vi "Test UTF Job.vi"() -> ()   [LabVIEW 2014]
uses:
  Core/LabVIEW CI Service/Extensions/Run UTF/Run UTF/Run UTF - STYP.ctl
  Core/LabVIEW CI Service/Classes/Status Updater/Status Updater.lvclass/Status Updater.ctl
  Core/LabVIEW CI Service/Classes/Job/Job.lvclass/Job.ctl
  Core/LabVIEW CI Service/Extensions/Run UTF/Run UTF/Run UTF.lvclass
  Core/LabVIEW CI Service/Classes/Status Updater/Status Updater.lvclass
  Core/LabVIEW CI Service/Classes/Job/Job.lvclass
panel:
  in  "Workspace Path":path=path "P:/alsmith/Sales/users/ACS/LabVIEW Continuous Integration/Jenkins Sample Project/Run VI Golden DUT.vi"
  out "Results":T1 {"Status" items=["Service Error"=504, "Abort"=503, "Fail"=500, "Pass"=200]}
  out "Steps":string[](array[string])
  out "Progress Percents":u32[](array[numeric])
  in  "VI Path":path=path "P:/alsmith/Sales/users/ACS/LabVIEW Continuous Integration/Jenkins Sample Project/Run VI Golden DUT.vi"
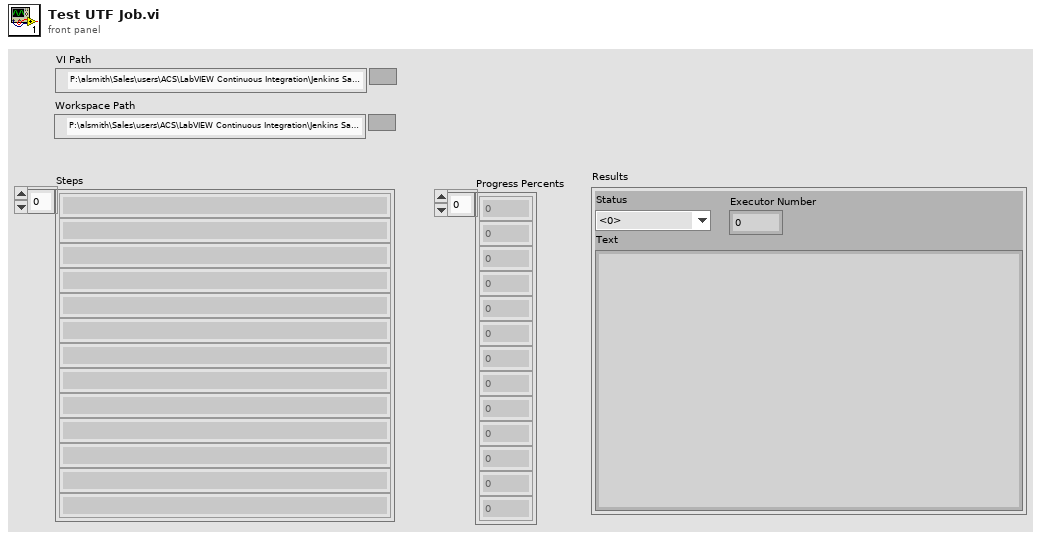
[diagram p1: front panel]
types:
  T1 = cluster{"Status":u16, "Text":string, "Executor Number":i32}
  T2 = typedef "Run UTF - STYP.ctl" = cluster{"Project Path":string}
  T3 = cluster{"Event Registration Refnum":refnum<event-registration>, "Event Registration Refnum":refnum<event-registration>}
  T4 = typedef "Job Results - STYP.ctl" = cluster{"Status":u16, "Text":string, "Executor Number":i32}
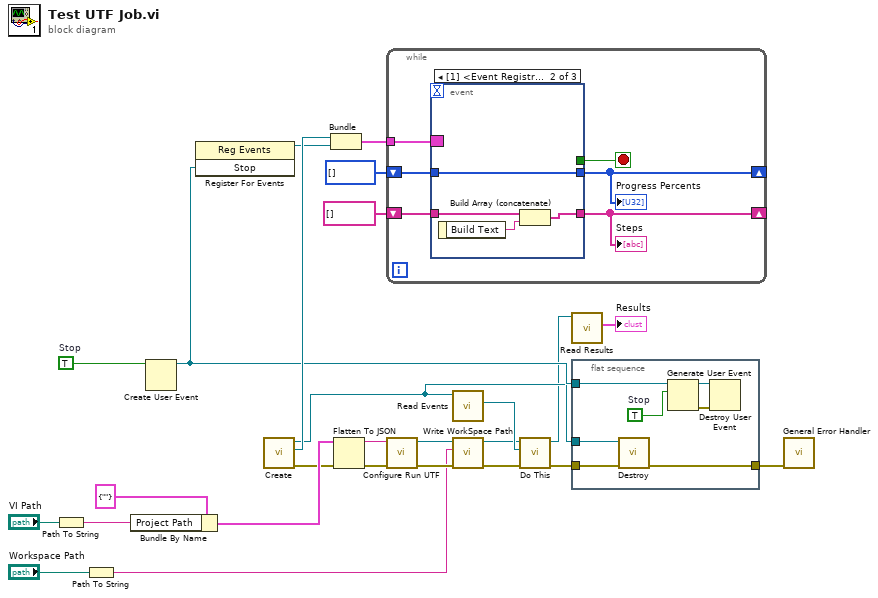
[diagram p0: block diagram]
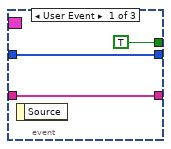
[diagram p2: hidden frame]
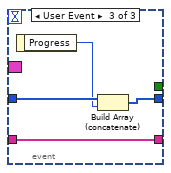
[diagram p3: hidden frame]
diagram:
  w22 = TRUE  # Stop
  n1 = Path To String(path="VI Path") -> (string=w25:string)
  n2 = Path To String(path="Workspace Path") -> (string=w1:string)
  n3 = Bundle By Name(cluster=T2 {"Project Path"=""} ("Run UTF"), "Project Path"=w25) -> (w26:T2)
  n4 = Create User Event(user event datatype=w22) -> (user event=w18:refnum<user-event>)  [unwired: 1 in, 1 out]
  n5 = register-events(w18) -> (reference out=w19:refnum<event-registration>)  [unwired: 2 in, 1 out]
  n6 = call "Create.vi"() -> ("error out"=w23:errorcluster, "Event Registration Refnum"=w21:refnum<event-registration>, "Status Updater out"=w13:refnum<class "Status Updater.lvclass">)  [unwired: 9 in]
  n7 = Bundle("Event Registration Refnum"=w21, "Event Registration Refnum"=w19) -> (w20:T3)  [unwired: 1 in]
  n8 = Flatten To JSON(anything=w26, error in (no error)=w23) -> (JSON string=w11:string, 11:w12:errorcluster)  [unwired: 1 in]
  n9 = while {
    tunnel: w20 -> [w32]
    shift-right: [w28] -> _
    shift-left: string[] [] -> [w30]
    shift-right: [w27] -> _
    shift-left: u32[] [] -> [w29]
    stop <- w31 stop-if-true
    n10 = event shown="[1] <Event Registration Refnum.Events.Build Text>: User Event" {
      selector: w32 -> [_ _ _]
      dyn-events: _ -> [_ _ _]
      timeout: _ -> [_ _ _]
      tunnel: [TRUE _ _] -> w31
      tunnel: w30 -> [w34 w39 w43]
      tunnel: [w34 w38 w43] -> w28
      tunnel: w29 -> [w33 w36 w42]
      tunnel: [w33 w36 w41] -> w27
      event User Event {
        n11 = event-data() -> ()  [unwired: 1 in, 1 out]
      }
      event User Event {
        n12 = event-data() -> ("Build Text"=w37:string)  [unwired: 1 in]
        n13 = Build Array (concatenate)(w39, w37) -> (w38:string[])
      }
      event User Event {
        n14 = event-data() -> ("Progress"=w40:u32)  [unwired: 1 in]
        n15 = Build Array (concatenate)(w42, w40) -> (w41:u32[])
      }
    }
    "Steps" <- w28
    "Progress Percents" <- w27
  }
  n16 = call "Configure Run UTF.vi"("error in (no error)"=w12, "JSON string"=w11) -> ("error out"=w4:errorcluster, "Run UTF.lvclass"=w6:refnum<class "Run UTF.lvclass">)  [unwired: 8 in]
  n17 = call "Read Events.vi"("Status Updater in"=w13) -> ("Status Events"=w9:refnum<class "Status Events.lvclass">)  [unwired: 10 in]
  n18 = call "Write WorkSpace Path.vi"("error in (no error)"=w4, "WorkSpace Path"=w1, "Job in"=w6) -> ("error out"=w3:errorcluster, "Job out"=w5:refnum<class "Run UTF.lvclass">)  [unwired: 7 in]
  n19 = call-dynamic "Do This.vi"("error in (no error)"=w3, "Status Events"=w9, "Run UTF in"=w5) -> ("error out"=w7:errorcluster, "Run UTF out"=w8:refnum<class "Run UTF.lvclass">)  [unwired: 7 in]
  n20 = call "Read Results.vi"("Job in"=w8) -> ("Results"=→"Results":T4)  [unwired: 10 in]
  n21 = flat-sequence {
    tunnel: w13 -> [w50]
    tunnel: w7 -> [w49]
    tunnel: w18 -> [w47]
    tunnel: [w46] -> w15
    frame #0 {
      w48 = TRUE  # Stop
      n22 = call "Destroy.vi"("error in (no error)"=w49, "Status Updater in"=w50) -> ("error out"=w46:errorcluster)  [unwired: 9 in]
      n23 = Generate User Event(user event=w47, event data cluster=w48) -> (user event out=w44:refnum<user-event>, error out=w45:errorcluster)  [unwired: 2 in]
      n24 = Destroy User Event(user event=w44, error in=w45) -> ()  [unwired: 1 out]
    }
  }
  n25 = call <vilib>:"General Error Handler.vi"("error in (no error)"=w15) -> ()  [unwired: 10 in, 5 out]
